vi "SSL Detection Frame Simple Estimator Cameras.vi"(5 "Estimador":T1, 7 "Enable":bool, 8 "ignora esquerda?":bool=TRUE, 9 "ignora lado?":bool=TRUE, 10 "Field Size":T2, 11 "Detection Frame In":T3 {"robots_blue"."height" format="%+4.3f"; "robots_blue"."pixel_y" format="%+4.3f"; "robots_blue"."pixel_x" format="%+4.3f"; "robots_blue"."orientation" format="%+4.3f"; "robots_blue"."y" format="%+4.3f"; "robots_blue"."confidence" format="%4.3f"; "robots_blue"."x" format="%+4.3f"; "robots_yellow"."height" format="%+4.3f"; "robots_yellow"."pixel_y" format="%+4.3f"; "robots_yellow"."pixel_x" format="%+4.3f"; "robots_yellow"."orientation" format="%+4.3f"; "robots_yellow"."y" format="%+4.3f"; "robots_yellow"."confidence" format="%4.3f"; "robots_yellow"."x" format="%+4.3f"}) -> (2 "Field Size Out":T2, 3 "Detection Frame Out":T3 {"robots_blue"."height" format="%+4.3f"; "robots_blue"."pixel_y" format="%+4.3f"; "robots_blue"."pixel_x" format="%+4.3f"; "robots_blue"."orientation" format="%+4.3f"; "robots_blue"."y" format="%+4.3f"; "robots_blue"."confidence" format="%4.3f"; "robots_blue"."x" format="%+4.3f"; "robots_yellow"."height" format="%+4.3f"; "robots_yellow"."pixel_y" format="%+4.3f"; "robots_yellow"."pixel_x" format="%+4.3f"; "robots_yellow"."orientation" format="%+4.3f"; "robots_yellow"."y" format="%+4.3f"; "robots_yellow"."confidence" format="%4.3f"; "robots_yellow"."x" format="%+4.3f"})   [LabVIEW 2016]
uses:
  SSL Detection Frame.ctl
  SSL Detection Robot.ctl
  <vilib>/Analysis/Matrix/Datatypes/RealMatrix.ctl
  SSL Detection Ball.ctl
  Filters/Estimadores.ctl
  <vilib>/Analysis/Matrix/NI_Matrix.lvlib
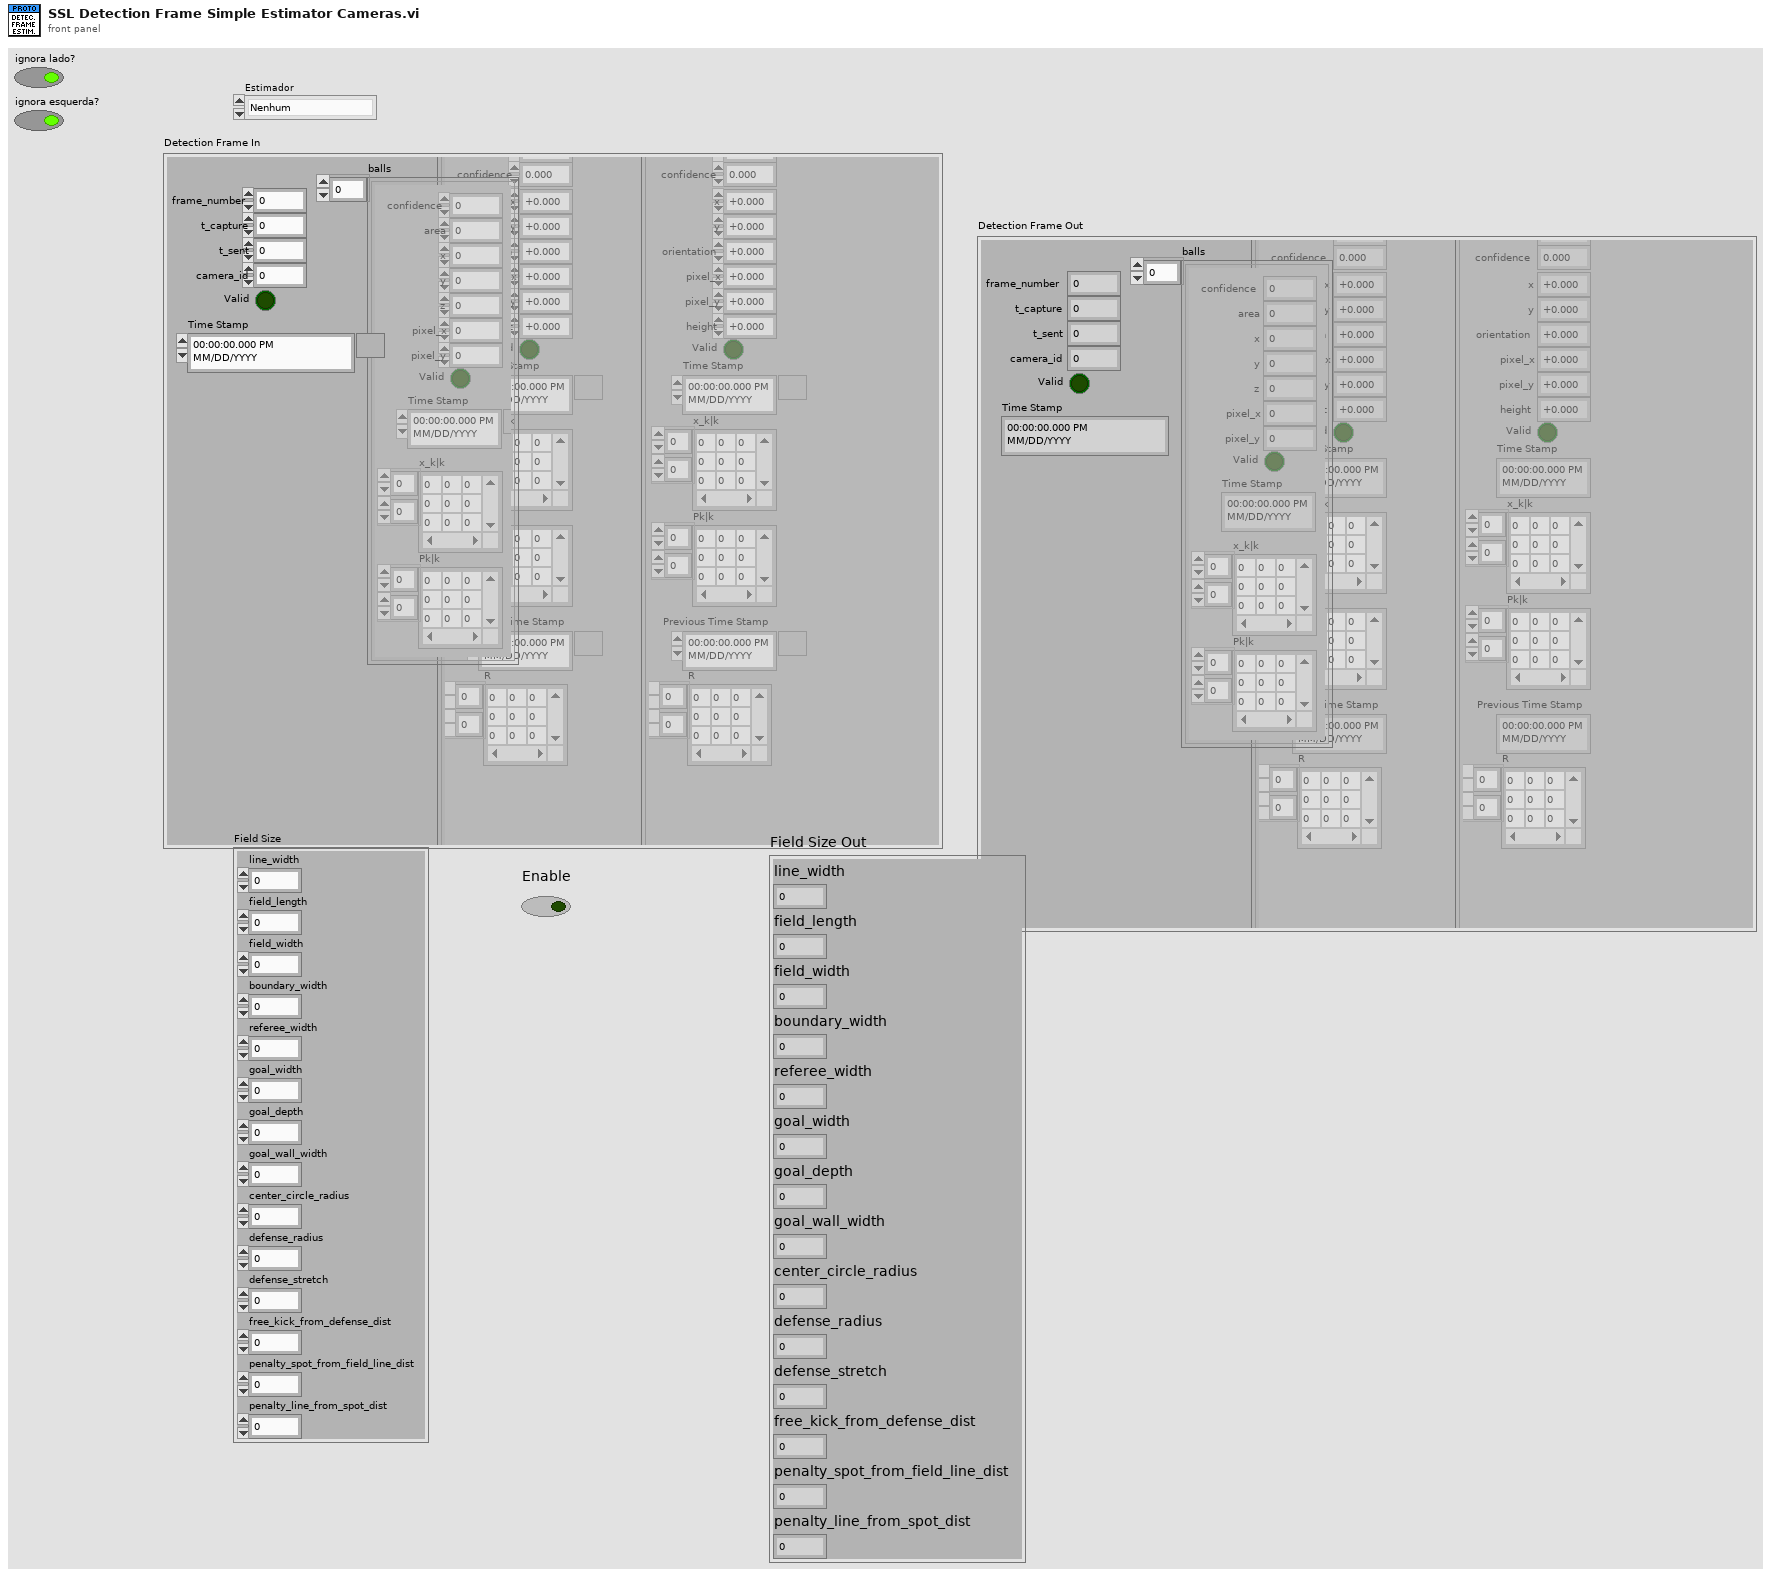
[diagram p1: front panel]
types:
  T1 = typedef "Estimadores.ctl" = enum16{"Nenhum", "Simples", "Kalman"}
  T2 = cluster{"line_width":u32, "field_length":u32, "field_width":u32, "boundary_width":u32, "referee_width":u32, "goal_width":u32, "goal_depth":u32, "goal_wall_width":u32, "center_circle_radius":u32, "defense_radius":u32, "defense_stretch":u32, "free_kick_from_defense_dist":u32, "penalty_spot_from_field_line_dist":u32, "penalty_line_from_spot_dist":u32}
  T3 = typedef "SSL Detection Frame.ctl" = cluster{"frame_number":u32, "t_capture":dbl, "t_sent":dbl, "camera_id":u32, "robots_yellow":T4[], "robots_blue":T4[], "balls":T6[], "Valid":bool, "Time Stamp":timestamp}
  T4 = typedef "SSL Detection Robot.ctl" = cluster{"x":sgl, "robot_id":u32, "confidence":sgl, "y":sgl, "orientation":sgl, "pixel_x":sgl, "pixel_y":sgl, "height":sgl, "Valid":bool, "Time Stamp":timestamp, "x_k|k":T5, "Pk|k":T5, "Previous Time Stamp":timestamp, "R":T5}
  T5 = typedef "NI_Matrix.lvlib/RealMatrix.ctl" = dbl[][]
  T6 = typedef "SSL Detection Ball.ctl" = cluster{"x":sgl, "area":u32, "confidence":sgl, "y":sgl, "z":sgl, "pixel_x":sgl, "pixel_y":sgl, "Valid":bool, "Time Stamp":timestamp, "x_k|k":T5, "Pk|k":T5}
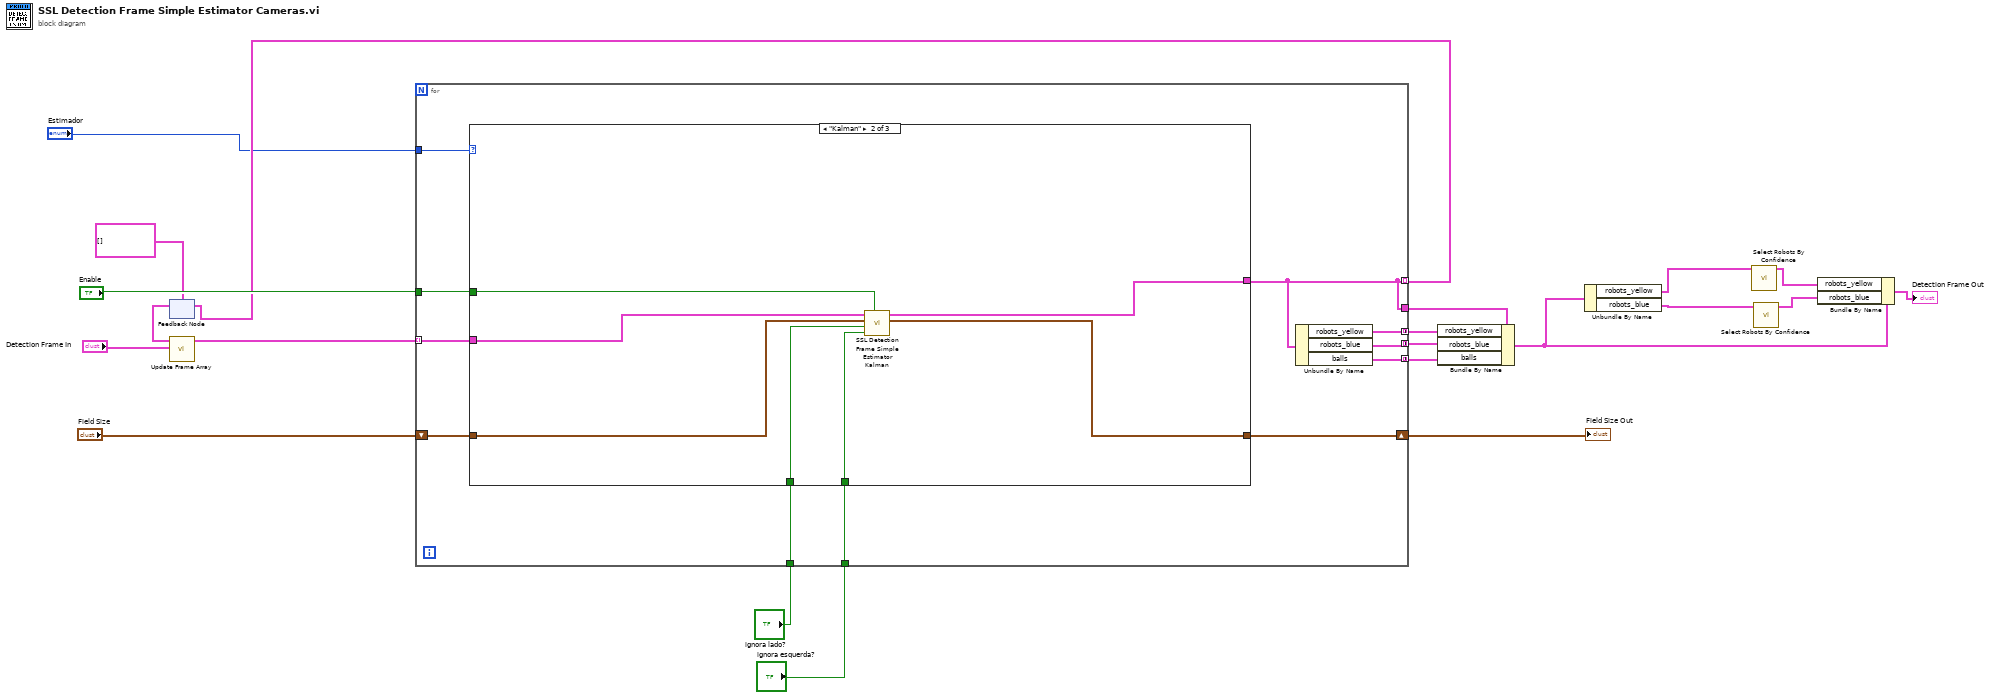
[diagram p0: block diagram]
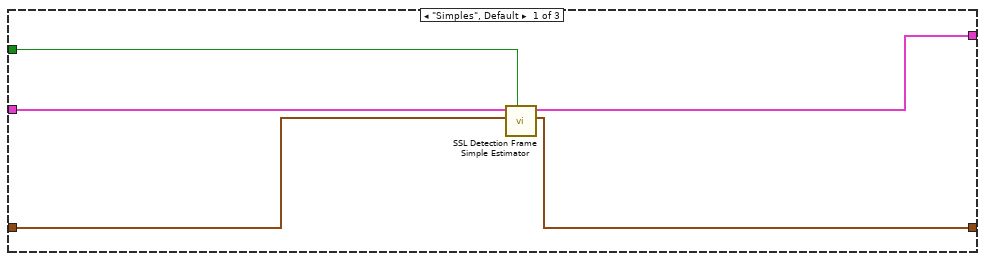
[diagram p2: hidden frame]
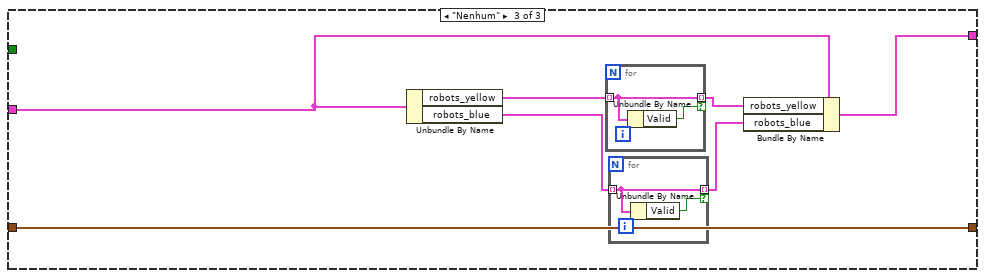
[diagram p3: hidden frame]
diagram:
  n1 = feedback #1(T3[] [] ("Detection Frame In out")) -> (w17:T3[])
  n2 = call "Update Frame Array.vi"("Detection Frame In"="Detection Frame In", "Detection Frame In 2"=w17) -> ("Detection Frame In out"=w18:T3[])  [unwired: 9 in]
  n3 = for {
    tunnel: [w24] -> w11 mode=indexing
    tunnel: "Estimador" -> [w30]
    tunnel: "Enable" -> [w29]
    tunnel: w18 -> [w28] mode=indexing
    shift-right: [w31] -> w20
    shift-left: "Field Size" -> [w32]
    tunnel: [w27] -> w14 mode=concatenating
    tunnel: [w26] -> w13 mode=concatenating
    tunnel: [w25] -> w12 mode=concatenating
    tunnel: [w24] -> w15
    tunnel: "ignora lado?" -> [w23]
    tunnel: "ignora esquerda?" -> [w22]
    n4 = case shown="\"Kalman\"" w30 {
      tunnel: [w33 w43 w47] -> w24
      tunnel: w28 -> [w37 w44 w49]
      tunnel: w29 -> [w36 w40 _]
      tunnel: w32 -> [w35 w42 w51]
      tunnel: [w34 w41 w51] -> w31
      tunnel: w23 -> [_ w39 _]
      tunnel: w22 -> [_ w38 _]
      frame "Simples", Default {
        n5 = call "SSL Detection Frame Simple Estimator.vi"("Enable"=w36, "Field Size"=w35, "Detection Frame In"=w37) -> ("Field Size Out"=w34:T2, "Detection Frame Out"=w33:T3)  [unwired: 7 in]
      }
      frame "Kalman" {
        n6 = call "SSL Detection Frame Simple Estimator Kalman.vi"("Enable"=w40, "ignora esquerda?"=w38, "ignora lado?"=w39, "Field Size"=w42, "Detection Frame In"=w44) -> ("Field Size Out"=w41:T2, "Detection Frame Out"=w43:T3)  [unwired: 5 in]
      }
      frame "Nenhum" {
        n7 = Unbundle By Name(w49) -> ("robots_yellow"=w50:T4[], "robots_blue"=w46:T4[])
        n8 = for {
          tunnel: w50 -> [w55] mode=indexing
          tunnel: [w55] -> w48 mode=indexing if=w54
          n9 = Unbundle By Name(w55) -> ("Valid"=w54:bool)
        }
        n10 = for {
          tunnel: w46 -> [w53] mode=indexing
          tunnel: [w53] -> w45 mode=indexing if=w52
          n11 = Unbundle By Name(w53) -> ("Valid"=w52:bool)
        }
        n12 = Bundle By Name(cluster=w49, "robots_yellow"=w48, "robots_blue"=w45) -> (w47:T3)
      }
    }
    n13 = Unbundle By Name(w24) -> ("robots_yellow"=w27:T4[], "robots_blue"=w26:T4[], "balls"=w25:T6[])
  }
  "Field Size Out" <- w20
  n14 = feedback-in #1(w11) -> ()
  n15 = Bundle By Name(cluster=w15, "robots_yellow"=w14, "robots_blue"=w13, "balls"=w12) -> (w8:T3)
  n16 = Unbundle By Name(w8) -> ("robots_yellow"=w4:T4[], "robots_blue"=w9:T4[])
  n17 = call "Select Robots By Confidence.vi"("robots_blue"=w4) -> ("Array"=w3:T4[])  [unwired: 10 in]
  n18 = call "Select Robots By Confidence.vi"("robots_blue"=w9) -> ("Array"=w7:T4[])  [unwired: 10 in]
  n19 = Bundle By Name(cluster=w8, "robots_yellow"=w3, "robots_blue"=w7) -> (→"Detection Frame Out":T3)
